vi "Load Confluence Connection Settings.vi"(8 "Error in":errorcluster caption="Error in (no error)", 11 "Settings Path":path) -> (0 "Error out":errorcluster, 1 "Loaded Default?":bool, 3 "Confluence Connection Settings":T1)   [LabVIEW 2023, in "VIDoc Printer - Confluence.lvlib" / "VIDoc Settings - Confluence.lvclass"]
uses:
  VIDoc Settings - Confluence.lvclass
  VIDoc Settings/VIDoc Settings.lvclass
  2067bb56-986f-4b99-9ebc-956c6fe73354.vi
  Confluence Connection Settings.ctl
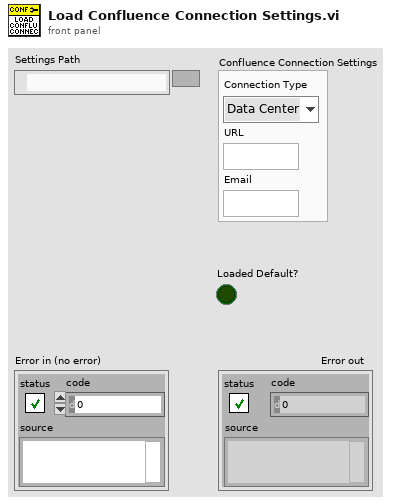
[diagram p1: front panel]
types:
  T1 = typedef "VIDoc Printer - Confluence.lvlib/VIDoc Settings - Confluence.lvclass/Confluence Connection Settings.ctl" = cluster{"Connection Type":enum16{"Data Center", "Cloud"}, "URL":string, "Email":string}
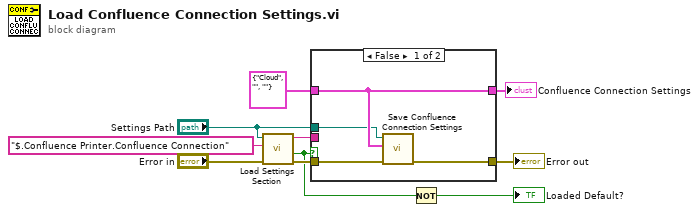
[diagram p0: block diagram]
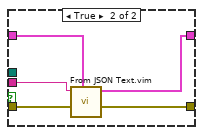
[diagram p2: hidden frame]
diagram:
  n1 = call "Load Settings Section.vi"("Error in"="Error in", "Section Name"="$.Confluence Printer.Confluence Connection", "JSON Settings Path"="Settings Path") -> ("Error out"=w8:errorcluster, "Found"=w3:bool, "JSON Object"=w7:string)  [unwired: 6 in]
  n2 = case shown="False" w3 {
    tunnel: w8 -> [w14 w19]
    tunnel: w7 -> [_ w18]
    tunnel: T1 {"Connection Type"=enum."Cloud", "URL"="", "Email"=""} ("Confluence Connection Settings") -> [w12 w17]
    tunnel: [w12 w16] -> w1
    tunnel: [w13 w15] -> w5
    tunnel: "Settings Path" -> [w11 _]
    frame False {
      n3 = call "Save Confluence Connection Settings.vi"("Error in"=w14, "Confluence Connection Settings"=w12, "Settings Path"=w11) -> ("Error out"=w13:errorcluster)  [unwired: 8 in]
    }
    frame True {
      n4 = call "From JSON Text.vim"("Data Type and Default Value"=w17, "error in (no error)"=w19, "JSON"=w18) -> ("error out"=w15:errorcluster, "Data out"=w16:T1)  [unwired: 7 in]
    }
  }
  "Error out" <- w5
  "Confluence Connection Settings" <- w1
  n5 = Not(x=w3) -> (.not. x?=→"Loaded Default?":bool)
